vi "GetCurrentProcessID.vi"(8 "Error In":errorcluster) -> (0 "Error Out":errorcluster, 3 "ProcessID":i32)   [LabVIEW 2021, in "Utilities.lvlib"]
uses:
  Utilities.lvlib
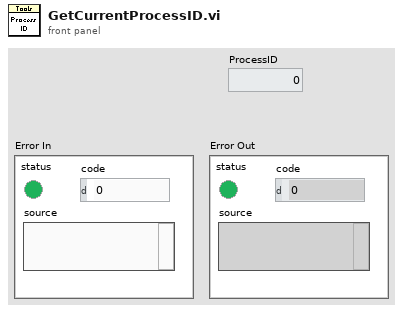
[diagram p1: front panel]
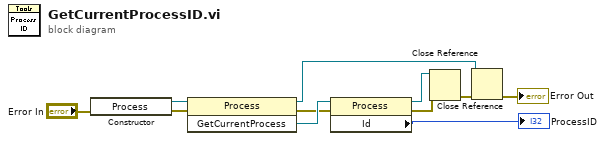
[diagram p0: block diagram]
diagram:
  n1 = constructor class="Process"(error in="Error In") -> (reference out=w7:refnum<k24>, error out=w6:errorcluster)  [unwired: 2 in, 1 out]
  n2 = invoke class="Process" method="GetCurrentProcess"(reference=w7, error in=w6) -> (reference out=w1:refnum<k24>, error out=w5:errorcluster, "GetCurrentProcess"=w8:refnum<k24>)  [unwired: 1 in]
  n3 = property class="Process"(reference=w8, error in=w5) -> (reference out=w4:refnum<k24>, error out=w3:errorcluster, "Id"=→"ProcessID":i32)
  n4 = Close Reference(reference=w4, error in (no error)=w3) -> (error out=w2:errorcluster)
  n5 = Close Reference(reference=w1, error in (no error)=w2) -> (error out=→"Error Out":errorcluster)
